vi "Conformity.vi"() -> (1 "整合后":T1(array[cluster]) {"MessageBuffer"."ID" format="%.0x"; "MessageBuffer"."DATA[0]" format="%.0x"}, 2 "时间段":u16[](array[numeric]))   [LabVIEW 2020]
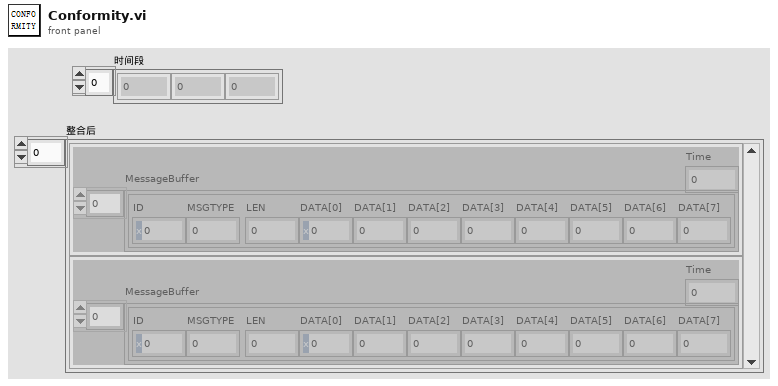
[diagram p1: front panel]
types:
  T1 = cluster{"Time":u16, "MessageBuffer":cluster{"ID":u32, "MSGTYPE":u8, "LEN":u8, "DATA[0]":u8, "DATA[1]":u8, "DATA[2]":u8, "DATA[3]":u8, "DATA[4]":u8, "DATA[5]":u8, "DATA[6]":u8, "DATA[7]":u8}[]}[]
  T2 = cluster{"ID":u32, "MSGTYPE":u8, "LEN":u8, "DATA[0]":u8, "DATA[1]":u8, "DATA[2]":u8, "DATA[3]":u8, "DATA[4]":u8, "DATA[5]":u8, "DATA[6]":u8, "DATA[7]":u8}
  T3 = cluster{"Time":u16, "MessageBuffer":cluster{"ID":u32, "MSGTYPE":u8, "LEN":u8, "DATA[0]":u8, "DATA[1]":u8, "DATA[2]":u8, "DATA[3]":u8, "DATA[4]":u8, "DATA[5]":u8, "DATA[6]":u8, "DATA[7]":u8}[]}
  T4 = cluster{"ID":u32, "MSGTYPE":u8, "LEN":u8, "DATA[0]":u8, "DATA[1]":u8, "DATA[2]":u8, "DATA[3]":u8, "DATA[4]":u8, "DATA[5]":u8, "DATA[6]":u8, "DATA[7]":u8}[]
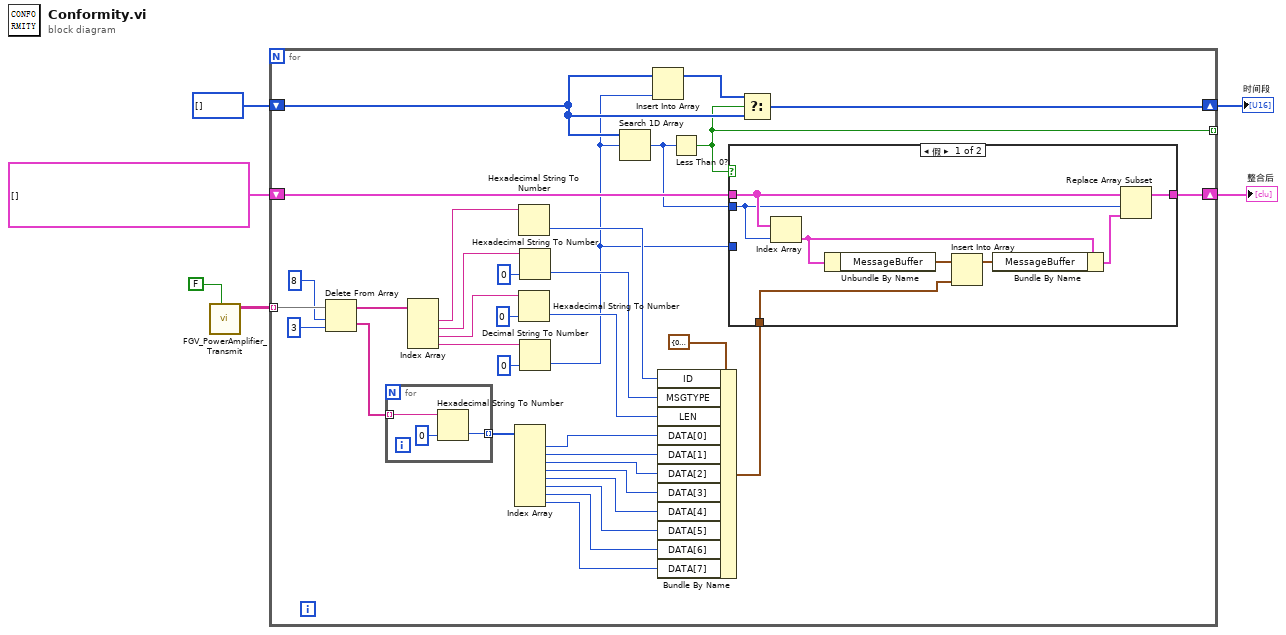
[diagram p0: block diagram]
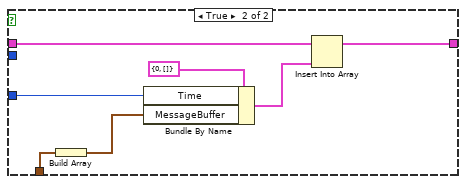
[diagram p2: hidden frame]
diagram:
  n1 = call "FGV_PowerAmplifier_Transmit.vi"("Write?"=FALSE) -> ("Transmit out"=w3:string[][])  [unwired: 9 in, 1 out]
  n2 = for {
    tunnel: w3 -> [w26] mode=indexing
    shift-right: [w38] -> w5
    shift-left: u16[] [] -> [w39]
    shift-right: [w36] -> w1
    shift-left: T1 [] ("整合后") -> [w37]
    tunnel: [w17] -> _ mode=indexing
    n3 = Delete From Array(array=w26, length=8 ("长度"), index=3 ("索引")) -> (deleted portion=w18:string[], array with subset deleted=w23:string[])
    n4 = for {
      tunnel: w18 -> [w42] mode=indexing
      tunnel: [w41] -> w15 mode=indexing
      n5 = Hexadecimal String To Number(string=w42, default (0uL)=u8 0 ("默认(0 I32)")) -> (number=w41:u8)  [unwired: 1 in, 1 out]
    }
    n6 = Index Array(array=w23) -> (element #1=w33:string, element #2=w31:string, element #3=w22:string, element #4=w19:string)  [unwired: 4 in]
    n7 = Index Array(array=w15) -> (element #1=w14:u8, element #2=w13:u8, element #3=w12:u8, element #4=w11:u8, element #5=w10:u8, element #6=w9:u8, element #7=w8:u8, element #8=w7:u8)  [unwired: 8 in]
    n8 = Hexadecimal String To Number(string=w33) -> (number=w32:u32)  [unwired: 2 in, 1 out]
    n9 = Hexadecimal String To Number(string=w22, default (0uL)=u8 0 ("默认(0 I32)")) -> (number=w29:u8)  [unwired: 1 in, 1 out]
    n10 = Hexadecimal String To Number(string=w31, default (0uL)=u8 0 ("默认(0 I32)")) -> (number=w30:u8)  [unwired: 1 in, 1 out]
    n11 = Decimal String To Number(string=w19, default (0L)=u16 0 ("默认(0 U32)")) -> (number=w20:u16)  [unwired: 1 in, 1 out]
    n12 = Search 1D Array(1D array=w39, element=w20) -> (index of element=w34:i32)  [unwired: 1 in]
    n13 = Insert Into Array(array=w39, new element=w20) -> (w40:u16[])  [unwired: 1 in]
    n14 = Bundle By Name(cluster=T2 {"ID"=0, "MSGTYPE"=0, "LEN"=0, "DATA[0]"=0, "DATA[1]"=0, "DATA[2]"=0, "DATA[3]"=0, "DATA[4]"=0, "DATA[5]"=0, "DATA[6]"=0, "DATA[7]"=0} ("MessageBuffer"), "ID"=w32, "MSGTYPE"=w30, "LEN"=w29, "DATA[0]"=w14, "DATA[1]"=w13, "DATA[2]"=w12, "DATA[3]"=w11, "DATA[4]"=w10, "DATA[5]"=w9, "DATA[6]"=w8, "DATA[7]"=w7) -> (w35:T2)
    n15 = Less Than 0?(x=w34) -> (x < 0?=w17:bool)
    n16 = case shown="假" w17 {
      tunnel: w37 -> [w50 w58]
      tunnel: [w51 w57] -> w36
      tunnel: w20 -> [_ w56]
      tunnel: w35 -> [w47 w54]
      tunnel: w34 -> [w49 _]
      frame False {
        n17 = Index Array(array=w50, index=w49) -> (element=w46:T3)
        n18 = Unbundle By Name(w46) -> ("MessageBuffer"=w48:T4)
        n19 = Insert Into Array(array=w48, new element=w47) -> (w45:T4)  [unwired: 1 in]
        n20 = Bundle By Name(cluster=w46, "MessageBuffer"=w45) -> (w44:T3)
        n21 = Replace Array Subset(array=w50, new element=w44, index=w49) -> (w51:T1)
      }
      frame True {
        n22 = Build Array(w54) -> (w52:T4)
        n23 = Bundle By Name(cluster=T3 {"Time"=0, "MessageBuffer"=[]} ("整合后"), "Time"=w56, "MessageBuffer"=w52) -> (w55:T3)
        n24 = Insert Into Array(array=w58, new element=w55) -> (w57:T1)  [unwired: 1 in]
      }
    }
    n25 = Select(t=w40, s=w17, f=w39) -> (s? t:f=w38:u16[])
  }
  "时间段" <- w5
  "整合后" <- w1
